vi "K6221_Check_Queue.vi"(7 "error in (no error)":errorcluster, 10 "queue":refnum<queue>) -> (0 "error out":errorcluster, 1 "Command (in)":T1, 3 "New Entries?":bool)   [LabVIEW 2019]
uses:
  K6221/K6221_Cluster.ctl
panel:
  out "Numeric":i32
  # "K 6221"
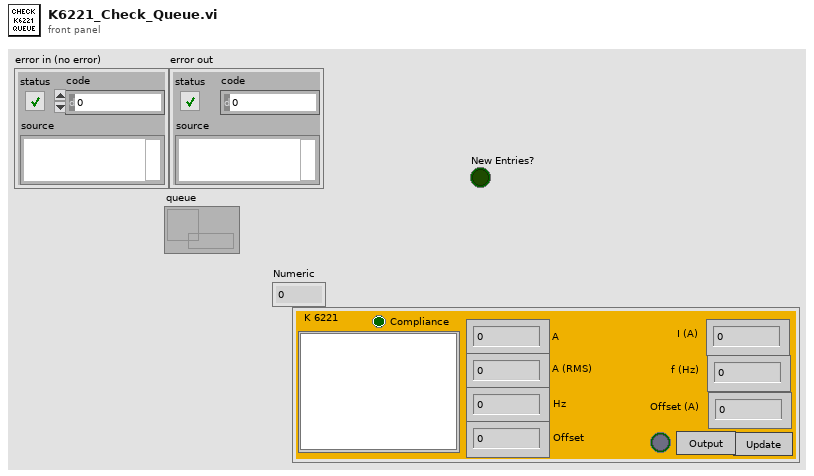
[diagram p1: front panel]
types:
  T1 = typedef "K6221_Cluster.ctl" = cluster{"Plot Window":dbl[][], "A":dbl, "A (RMS)":dbl, "Hz":dbl, "I (A)":dbl, "f (Hz)":dbl, "Update":bool, "Offset":dbl, "Offset (A)":dbl, "Compliance":bool, "Output":bool, "Output Status":bool}
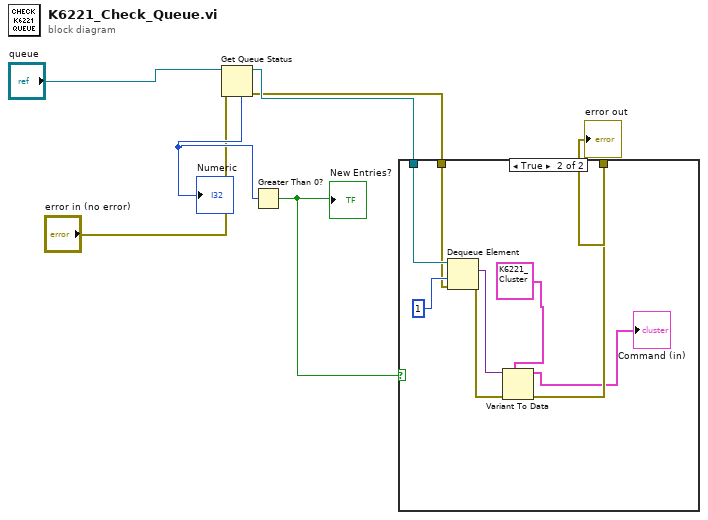
[diagram p0: block diagram]
diagram:
  n1 = Get Queue Status(queue="queue", error in (no error)="error in (no error)") -> (queue out=w6:refnum<queue>, error out=w4:errorcluster, # elements in queue=w7:i32)  [unwired: 1 in, 5 out]
  "Numeric" <- w7
  n2 = Greater Than 0?(x=w7) -> (x > 0?=w5:bool)
  "New Entries?" <- w5
  n3 = case shown="True" w5 {
    tunnel: w6 -> [_ w14]
    tunnel: w4 -> [w8 w13]
    tunnel: [w8 w11] -> w2
    frame False {
    }
    frame True {
      n4 = Dequeue Element(queue=w14, timeout in ms (-1)=1, error in (no error)=w13) -> (element=w15:variant, error out=w12:errorcluster)  [unwired: 2 out]
      n5 = Variant To Data(error in=w12, type=T1 {"Plot Window"=[], "A"=0.0, "A (RMS)"=0.0, "Hz"=0.0, "I (A)"=0.0, "f (Hz)"=0.0, "Update"=FALSE, "Offset"=0.0, "Offset (A)"=0.0, "Compliance"=FALSE, "Output"=FALSE, "Output Status"=FALSE} ("Command (in)"), Variant=w15) -> (data=→"Command (in)":T1, error out=w11:errorcluster)
    }
  }
  "error out" <- w2
